vi "randomize.vi"(11 "data bus":T1) -> (3 "data bus out":T1)   [LabVIEW 2024, in "IPE Optimization Tester.lvlib"]
uses:
  IPE Optimization Tester.lvlib
  data_bus--cluster.ctl
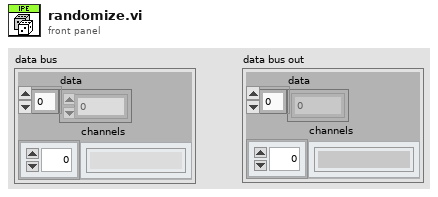
[diagram p1: front panel]
types:
  T1 = typedef "IPE Optimization Tester.lvlib/data_bus--cluster.ctl" = cluster{"data":dbl[], "channels":string[]}
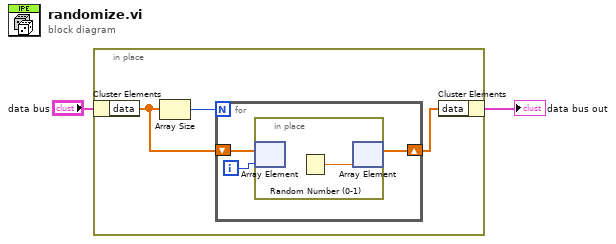
[diagram p0: block diagram]
diagram:
  n1 = in-place {
    n2 = in-place-cluster #1("data bus") -> ("data"=w4:dbl[])
    n3 = Array Size(array=w4) -> (size(s)=w5:i32)
    n4 = for {
      N: w5 -> [_]
      shift-right: [w6] -> w3
      shift-left: w4 -> [w8]
      i -> [w7]
      n5 = in-place {
        n6 = in-place-array #2(w8, w7) -> ()  [unwired: 1 out]
        n7 = Random Number (0-1)() -> (number: 0 to 1=w9:dbl)
        n8 = in-place-array #2(w9) -> (w6:dbl[])  [unwired: 1 out]
      }
    }
    n9 = in-place-cluster #1("data"=w3) -> (→"data bus out":T1)
  }
